vi "FeedbackDecode_LoadMSMSParams.vi"(2 "XMLFile":path=path "C:/Users/Administrator/Box/CNI/General/MSMS/Scenarios/MaleRight/Model/Prostheses/prosthesis.xml") -> (0 "ModelParams":T1={"ModelName"="MaleLeft", "Value"=[[0.002, -0.01, 0.0015], [0.0, 45.0, 0.0], [40.0, -40.0, 0.0], [0.0, 50.0, 0.0], [0.0, 75.0, 0.0], [0.0, -0.007, 0.005], [10.0, -13.0, 0.0], [0.0, 75.0, 0.0], [0.0, 75.0, 0.0], [0.0, 45.0, 0.0], [0.0, -0.005, 0.0055], [0.0, 75.0, 0.0], [0.0, 75.0, 0.0], [0.0, 45.0, 0.0], [0.0, 0.005, 0.0045], [-10.0, 10.0, 0.0], [0.0, 75.0, 0.0], [0.0, 75.0, 0.0], [0.0, 45.0, 0.0], [0.0006, 0.005, 0.0045], [-8.0, 15.0, 0.0], [0.0, 75.0, 0.0], [0.0, 75.0, 0.0], [0.0, 45.0, 0.0], [-0.03, -0.01, 0.015], [-45.0, 45.0, 0.0], [-45.0, 45.0, 0.0], [20.0, -20.0, 0.0]], "CompNames"=["\"ThumbSphere\"", "\"ThumbMeta\"", "\"ThumbSide\"", "\"ThumbKnuckle\"", "\"ThumbDIP\"", "\"IndexSphere\"", "\"IndexSide\"", "\"IndexKnuckle\"", "\"IndexPIP\"", "\"IndexDIP\"", "\"MiddleSphere\"", "\"MiddleKnuckle\"", "\"MiddlePIP\"", "\"MiddleDIP\"", "\"RingSphere\"", "\"RingSide\"", "\"RingKnuckle\"", "\"RingPIP\"", "\"RingDIP\"", "\"LittleSphere\"", "\"LittleSide\"", "\"LittleKnuckle\"", "\"LittlePIP\"", "\"LittleDIP\"", "\"WristSphere\"", "\"WristRoll\"", "\"WristPitch\"", "\"WristYaw\""]})   [LabVIEW 2020]
panel:
  in  "ParamsArray":T2(array[cluster])=[{"ModelName"="MaleLeft", "Value"=[[0.002, -0.01, 0.0015], [0.0, 45.0, 0.0], [20.0, -60.0, 0.0], [0.0, 50.0, 0.0], [0.0, 75.0, 0.0], [0.0, -0.007, 0.005], [10.0, -13.0, 0.0], [0.0, 75.0, 0.0], [0.0, 75.0, 0.0], [0.0, 45.0, 0.0], [0.0, -0.005, 0.0055], [0.0, 75.0, 0.0], [0.0, 75.0, 0.0], [0.0, 45.0, 0.0], [0.0, -0.005, 0.0045], [-10.0, 10.0, 0.0], [0.0, 75.0, 0.0], [0.0, 75.0, 0.0], [0.0, 45.0, 0.0], [0.0006, -0.005, 0.0045], [-8.0, 15.0, 0.0], [0.0, 75.0, 0.0], [0.0, 75.0, 0.0], [0.0, 45.0, 0.0], [-0.03, -0.01, 0.015], [-45.0, 45.0, 0.0], [-45.0, 45.0, 0.0], [20.0, -20.0, 0.0]], "CompNames"=["\"ThumbSphere\"", "\"ThumbMeta\"", "\"ThumbSide\"", "\"ThumbKnuckle\"", "\"ThumbDIP\"", "\"IndexSphere\"", "\"IndexSide\"", "\"IndexKnuckle\"", "\"IndexPIP\"", "\"IndexDIP\"", "\"MiddleSphere\"", "\"MiddleKnuckle\"", "\"MiddlePIP\"", "\"MiddleDIP\"", "\"RingSphere\"", "\"RingSide\"", "\"RingKnuckle\"", "\"RingPIP\"", "\"RingDIP\"", "\"LittleSphere\"", "\"LittleSide\"", "\"LittleKnuckle\"", "\"LittlePIP\"", "\"LittleDIP\"", "\"WristSphere\"", "\"WristRoll\"", "\"WristPitch\"", "\"WristYaw\""]}, {"ModelName"="MaleRight", "Value"=[[-0.01, -0.0075, 0.0], [-30.0, 45.0, 0.0], [0.0, -80.0, 0.0], [-25.0, 25.0, 0.0], [0.0, 75.0, 0.0], [0.0, -0.005, -0.0075], [10.0, -13.0, 0.0], [0.0, 75.0, 0.0], [0.0, 75.0, 0.0], [0.0, 45.0, 0.0], [0.0, -0.005, -0.0075], [0.0, 75.0, 0.0], [0.0, 75.0, 0.0], [0.0, 45.0, 0.0], [0.0, -0.005, -0.0075], [-10.0, 10.0, 0.0], [0.0, 75.0, 0.0], [0.0, 75.0, 0.0], [0.0, 45.0, 0.0], [0.0, -0.005, -0.0075], [-8.0, 15.0, 0.0], [0.0, 75.0, 0.0], [0.0, 75.0, 0.0], [0.0, 45.0, 0.0], [-0.04, -0.01, -0.017], [-45.0, 45.0, 0.0], [-45.0, 45.0, 0.0], [20.0, -20.0, 0.0]], "CompNames"=["\"ThumbSphere\"", "\"ThumbMeta\"", "\"ThumbSide\"", "\"ThumbKnuckle\"", "\"ThumbDIP\"", "\"IndexSphere\"", "\"IndexSide\"", "\"IndexKnuckle\"", "\"IndexPIP\"", "\"IndexDIP\"", "\"MiddleSphere\"", "\"MiddleKnuckle\"", "\"MiddlePIP\"", "\"MiddleDIP\"", "\"RingSphere\"", "\"RingSide\"", "\"RingKnuckle\"", "\"RingPIP\"", "\"RingDIP\"", "\"LittleSphere\"", "\"LittleSide\"", "\"LittleKnuckle\"", "\"LittlePIP\"", "\"LittleDIP\"", "\"WristSphere\"", "\"WristRoll\"", "\"WristPitch\"", "\"WristYaw\""]}]
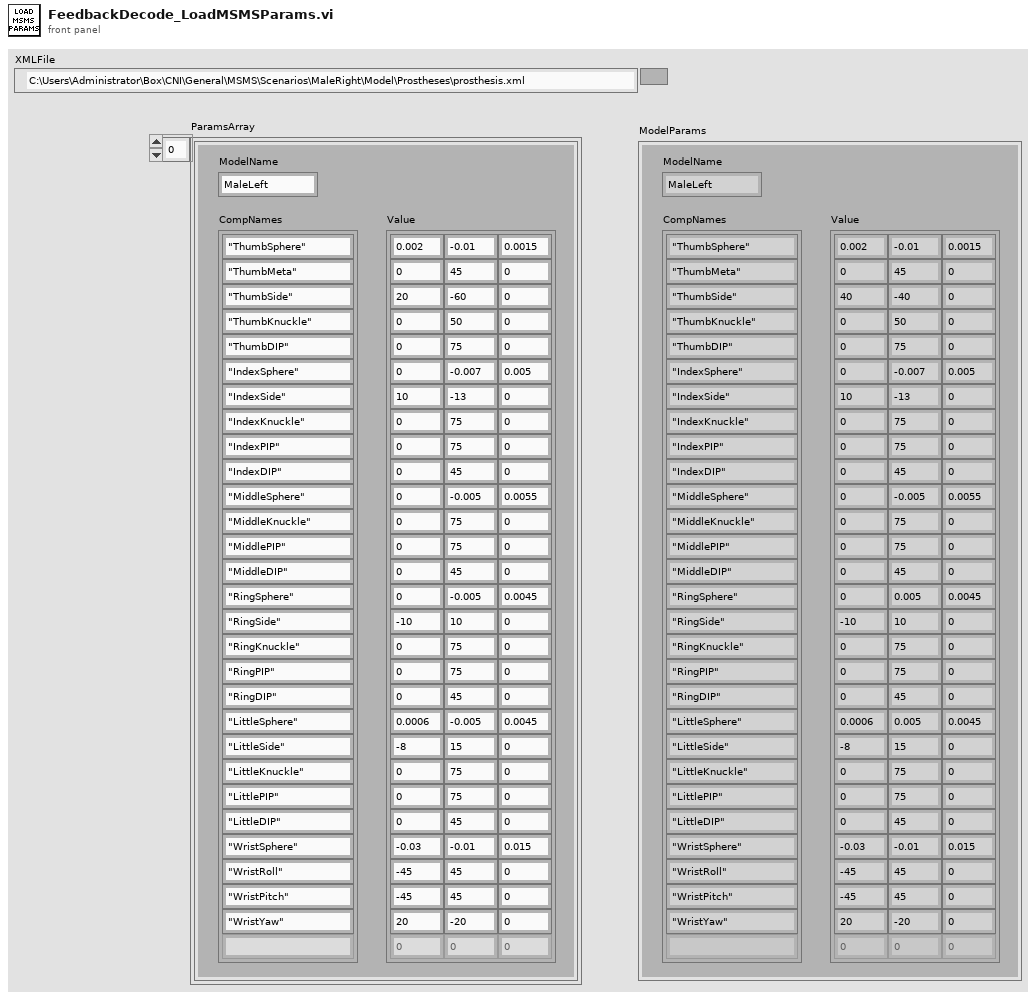
[diagram p1: front panel]
types:
  T1 = cluster{"ModelName":string, "Value":dbl[][], "CompNames":string[]}
  T2 = cluster{"ModelName":string, "Value":dbl[][], "CompNames":string[]}[]
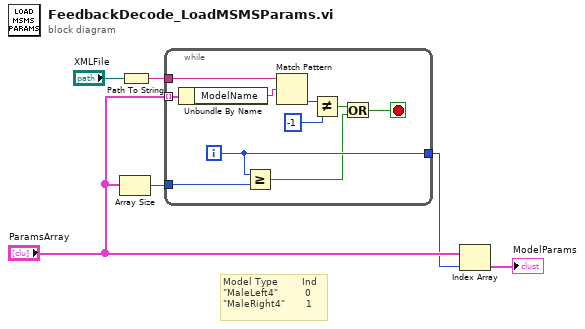
[diagram p0: block diagram]
diagram:
  # "Model Type        Ind\n\"MaleLeft4\"         0\n\"MaleRight4\"       1"
  n1 = Array Size(array="ParamsArray") -> (size(s)=w2:i32)
  n2 = Path To String(path="XMLFile") -> (string=w4:string)
  n3 = while {
    tunnel: w4 -> [w16]
    tunnel: "ParamsArray" -> [w15] mode=indexing
    tunnel: [w11] -> w1
    tunnel: w2 -> [w7]
    i -> [w11]
    stop <- w8 stop-if-true
    n4 = Unbundle By Name(w15) -> ("ModelName"=w14:string)
    n5 = Greater Or Equal?(x=w11, y=w7) -> (x >= y?=w9:bool)
    n6 = Match Pattern(string=w16, regular expression=w14) -> (offset past match=w12:i32)  [unwired: 1 in, 3 out]
    n7 = Not Equal?(x=w12, y=-1) -> (x != y?=w10:bool)
    n8 = Or(x=w10, y=w9) -> (x .or. y?=w8:bool)
  }
  n9 = Index Array(array="ParamsArray", index=w1) -> (element=→"ModelParams":T1)
